vi "IMU_Read_IDENT.vi"(8 "error in (no error)":errorcluster caption="Fehler (Eingang, kein Fehler)", 10 "VISA resource name IN":refnum<visa-resource-name>, 11 "MultiWii Data Cluster 2":refnum<vi>) -> (0 "error out":errorcluster caption="Fehler (Ausgang)", 2 "VISA resource name OUT":refnum<visa-resource-name>)   [LabVIEW 2017]
uses:
  IMU_Data_Cluster.ctl
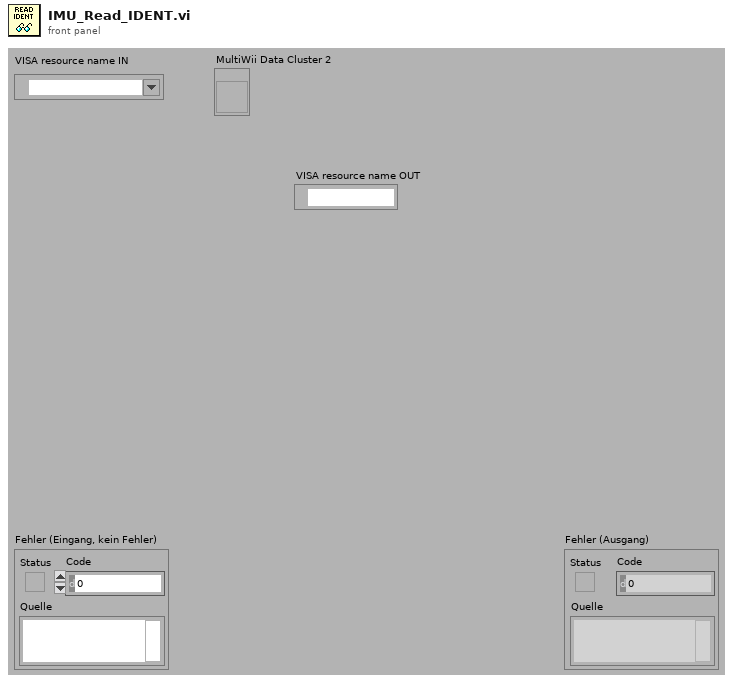
[diagram p1: front panel]
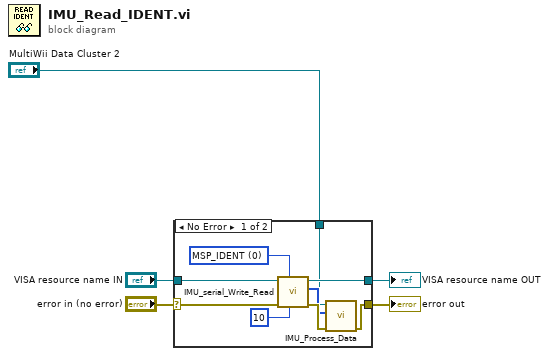
[diagram p0: block diagram]
diagram:
  n1 = case shown="No Error" "error in (no error)" {
    selector: "error in (no error)" -> [w8 w15]
    tunnel: "VISA resource name IN" -> [w14 w16]
    tunnel: [w11 w16] -> w4
    tunnel: [w10 w15] -> w3
    tunnel: "MultiWii Data Cluster 2" -> [w6 _]
    frame No Error {
      w9 = u16 0 items=["MSP_IDENT", "MSP_STATUS", "MSP_RAW_IMU", "MSP_RAW_GPS", "MSP_ATTITUDE", "MSP_ALTITUDE", "MSP_ACC_CALIBRATION", "MSP_MAG_CALIBRATION"] ("Command Selection")
      n2 = call "IMU_serial_Write_Read.vi"("Delay (ms)"=u32 10, "Command Selection"=w9, "error in (no error)"=w8, "VISA resource name IN"=w14) -> ("error IO"=w13:errorcluster, "Received Raw Data Byte-Array U8"=w12:u8[], "VISA resource name OUT"=w11:refnum<visa-resource-name>)  [unwired: 5 in]
      n3 = call "IMU_Process_Data.vi"("error in (no error)"=w13, "Received Raw Data Byte-Array U8"=w12, "MultiWii Data Cluster 2"=w6) -> ("error out"=w10:errorcluster)  [unwired: 8 in]
    }
    frame Error {
    }
  }
  "VISA resource name OUT" <- w4
  "error out" <- w3
